vi "Complex QR Factorization.vi"(0 "A":T1, 1 "algorithm":enum32{"Householder"}(ring)) -> (2 "Q":T1, 3 "R":T1, 4 "error":i32)   [LabVIEW 2020, in "NI_AALPro.lvlib"]
doc: "LabVIEW no longer supports this VI. Use the QR Decomposition VI instead.\nPerforms the QR factorization of <B>A</B>. You can use this polymorphic VI to perform QR factorization on a real matrix or a complex matrix. The data type you wire to the <B>A</B> input determines the polymorphic instance to use.\nQR factorization is also called orthogonal-triangular factorization. The QR Factorization VI factors matrix <B>A</B> so that <B>A</B> = <B>QR</B>. You can use QR factorization to solve linear systems with more equations than unknowns."
uses:
  NI_AALPro.lvlib
  ComplexMatrix.ctl
  <resource>/lvanlys.dll
  NI_Matrix.lvlib
panel:
  # "Complex QR Factorization"
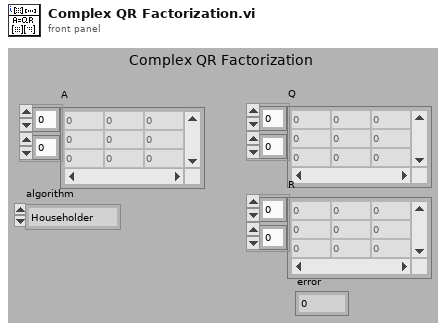
[diagram p1: front panel]
types:
  T1 = typedef "NI_Matrix.lvlib/ComplexMatrix.ctl" = cdb[][]
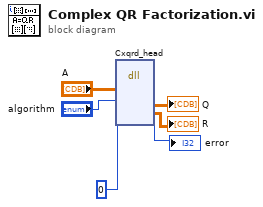
[diagram p0: block diagram]
diagram:
  n1 = dll-call lib="C:/Program Files (x86)/National Instruments/LabVIEW 2020/resource/lvanlys.*" fn="Cxqrd_head"("A"="A", "algorithm"="algorithm", 0) -> ("Q"=→"Q":T1, "R"=→"R":T1, →"error":i32)  [unwired: 8 in, 2 out]
